vi "Read Roles.vi"(8 "error in (no error)":errorcluster, 11 "TableWith2ndStrikerPlay in":refnum<class "TableWith2ndStrikerPlay.lvclass">) -> (0 "error out":errorcluster, 2 "Roles":T1, 3 "TableWith2ndStrikerPlay out":refnum<class "TableWith2ndStrikerPlay.lvclass">)   [LabVIEW 2018, in "TableWith2ndStrikerPlay.lvclass"]
uses:
  TableWith2ndStrikerPlay.lvclass
  TableFinalizerRole_class/TableFinalizerRole.lvclass
  TablerRole_class/TablerRole.lvclass
  PassObserverRole_class/PassObserverRole.lvclass
  TableWith2ndStrikerPlay.lvclass/TableWith2ndStrikerPlay.ctl
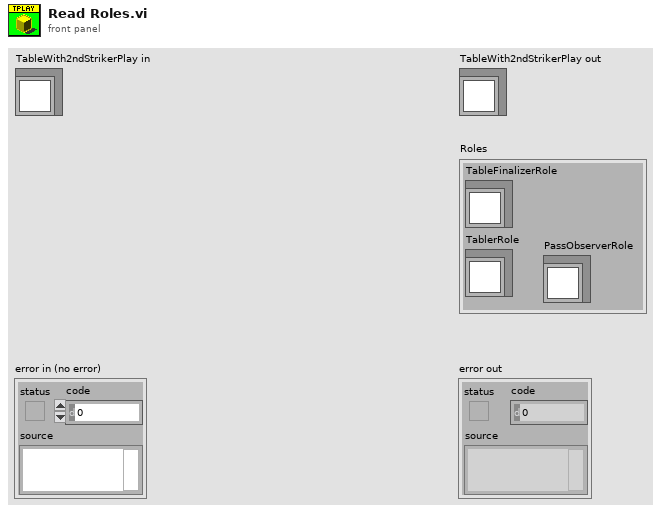
[diagram p1: front panel]
types:
  T1 = cluster{"TableFinalizerRole":refnum<class "TableFinalizerRole.lvclass">, "TablerRole":refnum<class "TablerRole.lvclass">, "PassObserverRole":refnum<class "PassObserverRole.lvclass">}
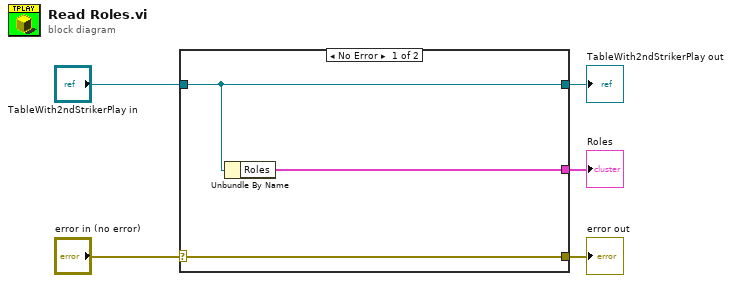
[diagram p0: block diagram]
diagram:
  n1 = case shown="No Error" "error in (no error)" {
    selector: "error in (no error)" -> [w8 w9]
    tunnel: [w8 w9] -> w4
    tunnel: [w7 w10] -> w2
    tunnel: "TableWith2ndStrikerPlay in" -> [w7 w10]
    tunnel: [w6 _] -> w1
    frame No Error {
      n2 = Unbundle By Name(w7) -> ("Roles"=w6:T1)
    }
    frame Error {
    }
  }
  "error out" <- w4
  "TableWith2ndStrikerPlay out" <- w2
  "Roles" <- w1
